vi "Pack for gRPC.vi"(8 "error in":errorcluster, 9 "configuration / results":enum16{"Configuration", "Results"}(ring), 10 "data value":variant, 11 "measurement customizations in":refnum<class "Measurement Plugin.lvclass">) -> (0 "error out":errorcluster, 2 "any":T1, 3 "measurement customizations out":refnum<class "Measurement Plugin.lvclass">)   [LabVIEW 2021, in "Crosstalkk_Audio ADC.lvlib" / "Measurement Plugin.lvclass"]
uses:
  Measurement Plugin.lvclass
  Measurement Plugin.lvclass/Measurement Plugin.ctl
  Measurement Configuration.ctl
  Crosstalkk_Audio ADC.lvlib
  Measurement Results.ctl
  a6012965-5700-4384-8228-972e71b6560c.vi
  2eca732d-dbaa-43bf-a7dd-ede2da65bc1b.vi
  <vilib>/MeasurementLink/MeasurementLink Measurement Server/Measurement Plugin Service/Measurement Plugin Service.lvclass
  C:/Program Files/National Instruments/LabVIEW 2021/vi.lib/MeasurementLink/MeasurementLink Measurement Server/Measurement Plugin Service/Measurement Plugin Service.lvclass
  C:/audio-adc-labview/source/crosstalk/crosstalk_Audio ADC/Advanced/Measurement Plugin.lvclass
  <vilib>/gRPC/LabVIEW gRPC Library/Shared/Any.ctl
  <vilib>/gRPC/LabVIEW gRPC Library/grpc-lvsupport-release.lvlib
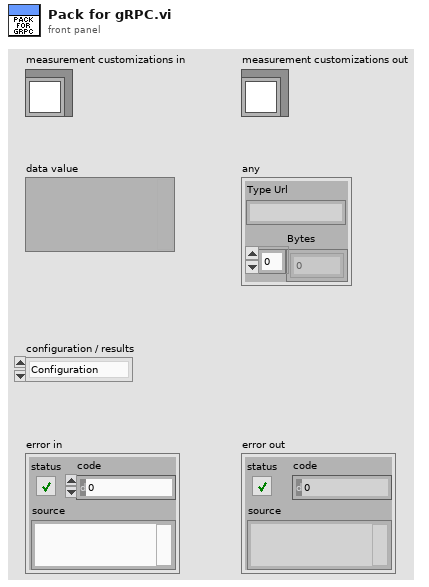
[diagram p1: front panel]
types:
  T1 = typedef "grpc-lvsupport-release.lvlib/Any.ctl" = cluster{"Type Url":string, "Bytes":u8[]}
  T2 = typedef "grpc-lvsupport-release.lvlib/grpcId.ctl" = u64
  T3 = typedef "Crosstalkk_Audio ADC.lvlib/Measurement Configuration.ctl" = cluster{"Weighting filter":string, "Full scale range":dbl, "Channel name":string, "Analog source resource name":string, "Frequency":dbl, "Amplitude":dbl, "Protocol capture resource name":string, "Data line":u32, "Interferer channel":u32, "Victim channel":u32, "Sample rate":dbl, "Measurement duration":dbl, "Frame sync edge for channel 0":u32, "Channel count per frame":u32, "Channel length":u32, "Bit depth":u32, "Channel 0 offset":u32, "Endiannes":u32, "Data justification":u32, "Frame length":u32, "Frame sync pulse width":u32, "Bit clock edge sync":u32}
  T4 = typedef "Crosstalkk_Audio ADC.lvlib/Measurement Results.ctl" = cluster{"Channel":string, "Crosstalk":dbl, "t0":dbl, "dt":dbl, "Time domain":dbl[], "Time domain size":i32, "f0":dbl, "df":dbl, "Spectrum":dbl[], "Spectrum size":i32}
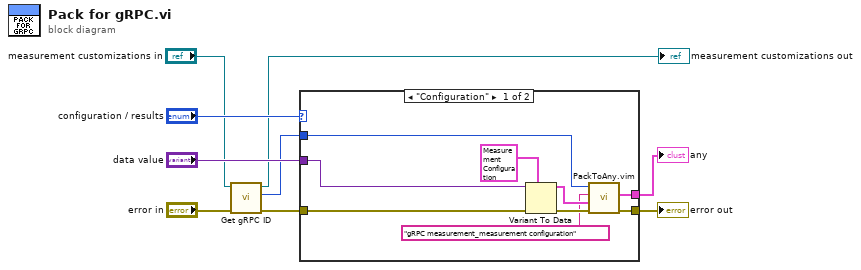
[diagram p0: block diagram]
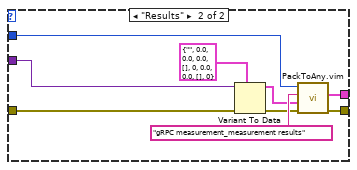
[diagram p2: hidden frame]
diagram:
  n1 = call <vilib>:"Get gRPC ID.vi"("error in"="error in", "measurement plugin service in"="measurement customizations in") -> ("error out"=w4:errorcluster, "gRPC ID"=w1:T2, "measurement plugin service out"=→"measurement customizations out":refnum<class "Measurement Plugin.lvclass">)  [unwired: 7 in]
  n2 = case shown="\"Configuration\"" "configuration / results" {
    tunnel: w4 -> [w18 w27]
    tunnel: "data value" -> [w17 w26]
    tunnel: w1 -> [w14 w22]
    tunnel: [w16 w24] -> w8
    tunnel: [w15 w23] -> w7
    frame "Configuration" {
      n3 = Variant To Data(error in=w18, type=T3 {"Weighting filter"="Linear", "Full scale range"=2.825, "Channel name"="", "Analog source resource name"="", "Frequency"=0.0, "Amplitude"=0.0, "Protocol capture resource name"="", "Data line"=0, "Interferer channel"=0, "Victim channel"=0, "Sample rate"=44100.0, "Measurement duration"=0.1, "Frame sync edge for channel 0"=1, "Channel count per frame"=2, "Channel length"=32, "Bit depth"=24, "Channel 0 offset"=1, "Endiannes"=0, "Data justification"=0, "Frame length"=64, "Frame sync pulse width"=32, "Bit clock edge sync"=1} ("measurement configuration"), Variant=w17) -> (data=w13:T3, error out=w12:errorcluster)
      n4 = call "PackToAny.vim"("error in"=w12, "Data To Pack"=w13, "Message Type"="gRPC measurement_measurement configuration", "gRPCid in"=w14) -> ("error out"=w16:errorcluster, "Any"=w15:T1)  [unwired: 5 in, 1 out]
    }
    frame "Results" {
      n5 = Variant To Data(error in=w27, type=T4 {"Channel"="", "Crosstalk"=0.0, "t0"=0.0, "dt"=0.0, "Time domain"=[], "Time domain size"=0, "f0"=0.0, "df"=0.0, "Spectrum"=[], "Spectrum size"=0} ("Measurement Results"), Variant=w26) -> (data=w20:T4, error out=w19:errorcluster)
      n6 = call "PackToAny.vim"("error in"=w19, "Data To Pack"=w20, "Message Type"="gRPC measurement_measurement results", "gRPCid in"=w22) -> ("error out"=w24:errorcluster, "Any"=w23:T1)  [unwired: 5 in, 1 out]
    }
  }
  "error out" <- w8
  "any" <- w7
